vi "FTP上传UI.vi"() -> ()   [LabVIEW 2016]
uses:
  <vilib>/FTP/NI_FTP.lvlib
panel:
  out "remote path":string
  out "temp path":path
  in  "上传版本txt":bool
  in  "read txt":bool
  in  "更新版本记录txt":string
  out "上传中":bool
  in  "remote port (21)":u16=21 caption="远程端口(21)"
  in  "password":string="std23506" caption="密码"
  in  "user":string="update" caption="用户"
  in  "host":string="27.154.58.30" caption="主机"
  in  "transfer spec":cluster{"remote path":string, "local path":path}={"remote path"="数据传输系统\\平台数据传输系统.exe\r\n", "local path"=path "C:/LabVIEW Project/builds/NEW平台数据传输系统/平台数据传输系统.exe"} caption="传输规范"
  in  "上传程序":bool
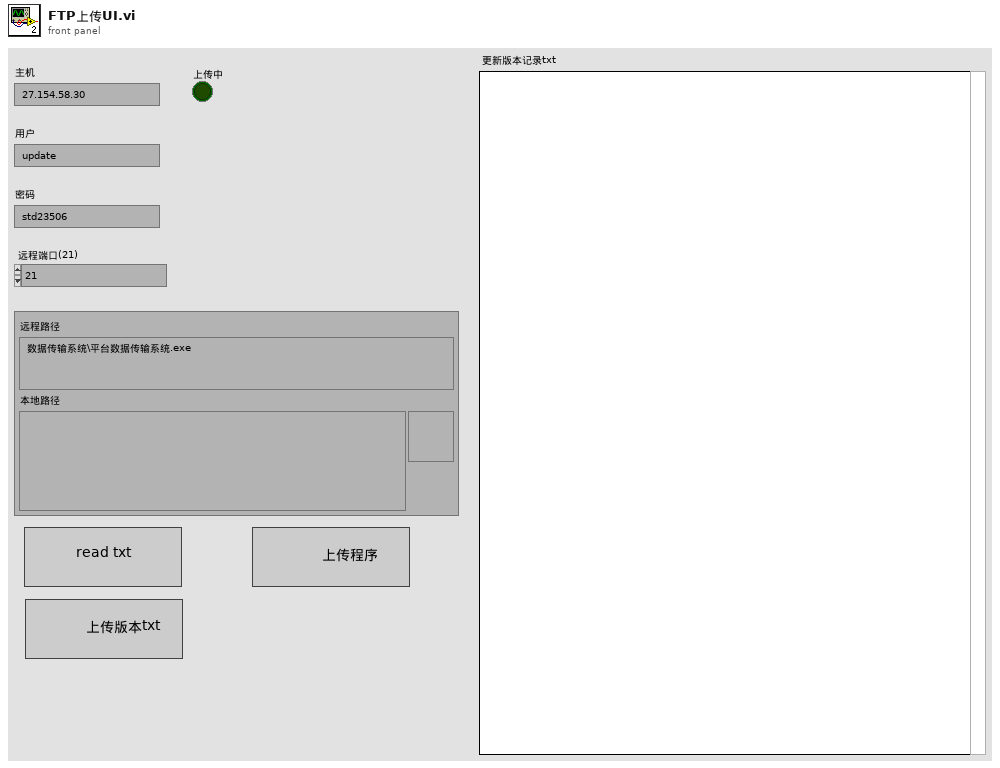
[diagram p1: front panel]
types:
  T1 = enum8{"Enabled", "Disabled", "Disabled and Grayed Out"}
  T2 = cluster{"remote path":string, "local path":path, "binary":bool}
  T3 = cluster{"remote path":string, "local path":path, "binary":bool}[]
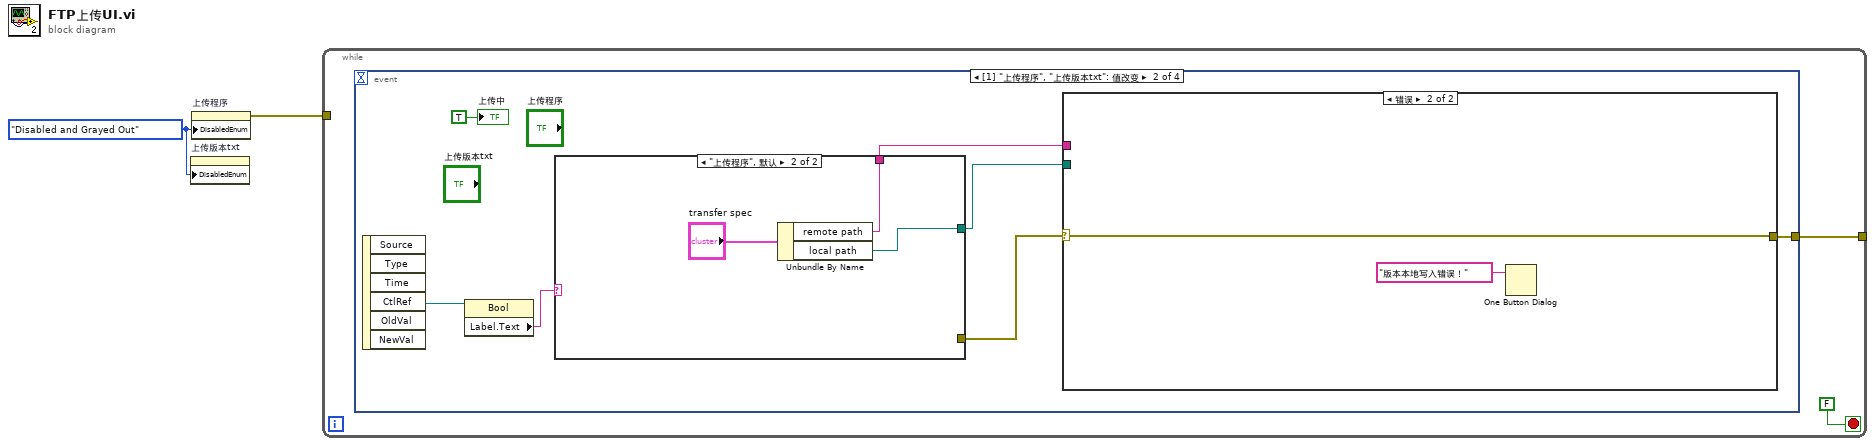
[diagram p0: block diagram]
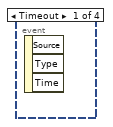
[diagram p2: hidden frame]
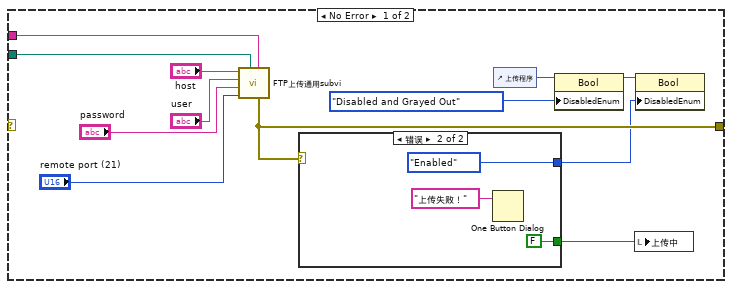
[diagram p3: hidden frame]
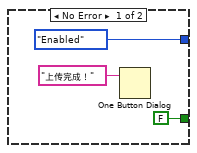
[diagram p4: hidden frame]
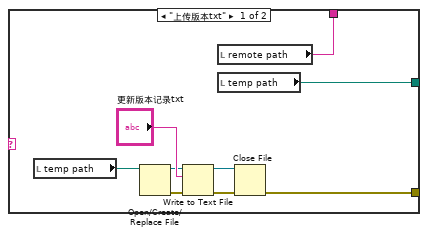
[diagram p5: hidden frame]
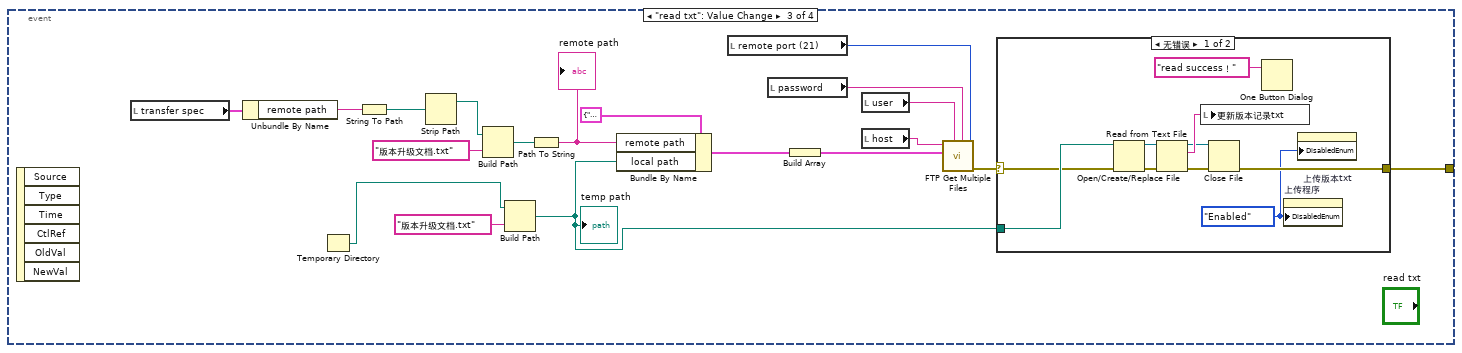
[diagram p6: hidden frame]
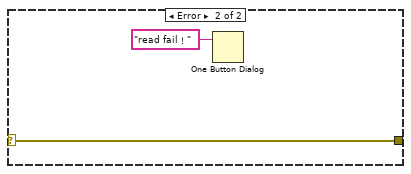
[diagram p7: hidden frame]
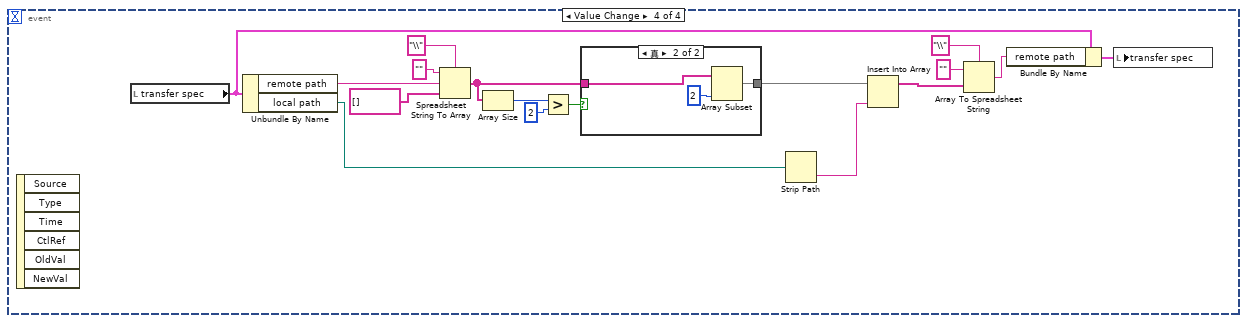
[diagram p8: hidden frame]
diagram:
  w1 = T1."Disabled and Grayed Out" ("禁用")
  n1 = property on="上传版本txt" class="Bool"("DisabledEnum"=w1) -> ()  [unwired: 2 in, 2 out]
  n2 = property on="上传程序" class="Bool"("DisabledEnum"=w1) -> (error out=w2:errorcluster)  [unwired: 2 in, 1 out]
  n3 = while {
    tunnel: [w4] -> _
    tunnel: w2 -> [_]
    stop <- FALSE stop-if-true
    n4 = event shown="[1] \"上传程序\", \"上传版本txt\": 值改变" {
      selector: _ -> [_ _ _ _]
      dyn-events: _ -> [_ _ _ _]
      timeout: _ -> [_ _ _ _]
      tunnel: [_ w11 w47 _] -> w4
      event Timeout {
        n5 = event-data() -> ()  [unwired: 1 in, 3 out]
      }
      event "上传程序", "上传版本txt": Value Change {
        n6 = event-data() -> ("CtlRef"=w9:refnum<vi>)  [unwired: 1 in, 5 out]
        n7 = property class="Bool"(reference=w9) -> ("Label.Text"=w8:string)  [unwired: 1 in, 2 out]
        n8 = case shown="\"上传程序\", 默认" w8 {
          tunnel: [w40 w42] -> w7
          tunnel: [w39 w41] -> w6
          tunnel: [w32 _] -> w5
          frame "上传版本txt" {
            n9 = local read "temp path"() -> (w38:path)
            n10 = Open/Create/Replace File(file path (use dialog)=w38) -> (refnum out=w36:refnum<file>, error out=w35:errorcluster)  [unwired: 5 in, 1 out]
            n11 = Write to Text File(file (use dialog)=w36, text="更新版本记录txt", error in=w35) -> (refnum out=w34:refnum<file>, error out=w33:errorcluster)  [unwired: 1 in, 1 out]
            n12 = local read "remote path"() -> (w40:string)
            n13 = local read "temp path"() -> (w39:path)
            n14 = Close File(refnum=w34, error in=w33) -> (error out=w32:errorcluster)  [unwired: 1 out]
          }
          frame "上传程序", Default {
            n15 = Unbundle By Name("transfer spec") -> ("remote path"=w42:string, "local path"=w41:path)
          }
        }
        n16 = case shown="错误" w5 {
          selector: w5 -> [_ w30]
          tunnel: [w19 w30] -> w11
          tunnel: w7 -> [w13 _]
          tunnel: w6 -> [w12 _]
          frame No Error {
            n17 = call "FTP上传通用subvi.vi"("remote path"=w13, "local path"=w12, "remote port (21)"="remote port (21)", "password"="password", "user"="user", "host"="host") -> ("error out"=w19:errorcluster)  [unwired: 4 in, 1 out]
            n18 = case shown="错误" w19 {
              tunnel: [FALSE FALSE] -> w18
              tunnel: [T1."Enabled" ("禁用") T1."Enabled" ("禁用")] -> w14
              frame No Error {
                n19 = One Button Dialog(message="上传完成！" ("消息")) -> ()  [unwired: 1 in, 1 out]
              }
              frame Error {
                n20 = One Button Dialog(message="上传失败！" ("消息")) -> ()  [unwired: 1 in, 1 out]
              }
            }
            n21 = control-ref of="上传程序"() -> (w17:refnum<vi>)
            n22 = property class="Bool"(reference=w17, "DisabledEnum"=T1."Disabled and Grayed Out" ("禁用")) -> (reference out=w15:refnum<vi>)  [unwired: 1 in, 1 out]
            n23 = local write "上传中"(w18) -> ()
            n24 = property class="Bool"(reference=w15, "DisabledEnum"=w14) -> ()  [unwired: 1 in, 2 out]
          }
          frame Error {
            n25 = One Button Dialog(message="版本本地写入错误！" ("消息")) -> ()  [unwired: 1 in, 1 out]
          }
        }
        "上传中" <- TRUE
      }
      event "read txt": Value Change {
        n26 = event-data() -> ()  [unwired: 1 in, 6 out]
        n27 = local read "transfer spec"() -> (w57:cluster{"remote path":string, "local path":path})
        n28 = Unbundle By Name(w57) -> ("remote path"=w56:string)
        n29 = Temporary Directory() -> (w45:path)
        n30 = String To Path(string=w56) -> (path=w55:path)
        n31 = Strip Path(path=w55) -> (stripped path=w54:path)  [unwired: 1 out]
        n32 = Build Path(base path=w54, name or relative path="版本升级文档.txt" ("名称或相对路径")) -> (appended path=w52:path)
        n33 = Build Path(base path=w45, name or relative path="版本升级文档.txt" ("名称或相对路径")) -> (appended path=w44:path)
        "temp path" <- w44
        n34 = Path To String(path=w52) -> (string=w51:string)
        "remote path" <- w51
        n35 = Bundle By Name(cluster=T2 {"remote path"="", "local path"=path "", "binary"=FALSE} ("元素"), "remote path"=w51, "local path"=w44) -> (w50:T2)
        n36 = local read "remote port (21)"() -> (w59:u16)
        n37 = local read "password"() -> (w60:string)
        n38 = Build Array(w50) -> (w49:T3)
        n39 = local read "user"() -> (w61:string)
        n40 = local read "host"() -> (w62:string)
        n41 = call <vilib>:"FTP Get Multiple Files.vi"("remote port (21)"=w59, "password"=w60, "user"=w61, "file specifications"=w49, "host"=w62) -> ("error out"=w48:errorcluster)  [unwired: 5 in, 1 out]
        n42 = case shown="无错误" w48 {
          selector: w48 -> [w64 w73]
          tunnel: w44 -> [w65 _]
          tunnel: [w66 w73] -> w47
          frame No Error {
            w63 = T1."Enabled" ("禁用")
            n43 = Open/Create/Replace File(file path (use dialog)=w65, error in=w64) -> (refnum out=w70:refnum<file>, error out=w69:errorcluster)  [unwired: 4 in, 1 out]
            n44 = Read from Text File(file (use dialog)=w70, error in=w69) -> (refnum out=w68:refnum<file>, text=w72:string, error out=w67:errorcluster)  [unwired: 2 in, 1 out]
            n45 = local write "更新版本记录txt"(w72) -> ()
            n46 = Close File(refnum=w68, error in=w67) -> (error out=w66:errorcluster)  [unwired: 1 out]
            n47 = One Button Dialog(message="read success！" ("消息")) -> ()  [unwired: 1 in, 1 out]
            n48 = property on="上传程序" class="Bool"("DisabledEnum"=w63) -> ()  [unwired: 2 in, 2 out]
            n49 = property on="上传版本txt" class="Bool"("DisabledEnum"=w63) -> ()  [unwired: 2 in, 2 out]
          }
          frame Error {
            n50 = One Button Dialog(message="read fail！" ("消息")) -> ()  [unwired: 1 in, 1 out]
          }
        }
      }
      event "transfer spec.local path": Value Change {
        n51 = event-data() -> ()  [unwired: 1 in, 6 out]
        n52 = local read "transfer spec"() -> (w90:cluster{"remote path":string, "local path":path})
        n53 = Unbundle By Name(w90) -> ("remote path"=w88:string, "local path"=w91:path)
        n54 = Spreadsheet String To Array(delimiter (Tab)="\\" ("分隔符(Tab)"), format string="" ("格式字符串"), spreadsheet string=w88, array type (2D Dbl)=string[] []) -> (array=w83:string[])
        n55 = Array Size(array=w83) -> (size(s)=w86:i32)
        n56 = Greater?(x=w86, y=2) -> (0:w84:bool)
        n57 = case shown="真" w84 {
          tunnel: w83 -> [w92 w94]
          tunnel: [w92 w93] -> w82
          frame False {
          }
          frame True {
            n58 = Array Subset(array=w94, length=2 ("长度")) -> (w93:string[])  [unwired: 1 in]
          }
        }
        n59 = Strip Path(path=w91) -> (name=w81:string)  [unwired: 1 out]
        n60 = Insert Into Array(array=w82, new element=w81) -> (w80:string[])  [unwired: 1 in]
        n61 = Array To Spreadsheet String(delimiter (Tab)="\\" ("分隔符(Tab)"), array=w80, 3:"" ("格式字符串")) -> (spreadsheet string=w79:string)
        n62 = Bundle By Name(cluster=w90, "remote path"=w79) -> (w89:cluster{"remote path":string, "local path":path})
        n63 = local write "transfer spec"(w89) -> ()
      }
    }
  }
